vi "Launch Client Handler Actor.vi"(6 "timeout ms (5000)":i32=5000, 8 "error in (no error)":errorcluster, 9 "Remote Address":string, 10 "WebSocket Connection in":refnum<k5>, 11 "Websocket Server in":refnum<class "Websocket Server.lvclass">) -> (0 "error out":errorcluster, 3 "Websocket Server out":refnum<class "Websocket Server.lvclass">)   [LabVIEW 2016, in "Stream Mediator.lvlib" / "Websocket Server.lvclass"]
doc: "--\nCopyright © 2017 Composed SystemsI All rights reserved.\n\nAuthor: Jon McBee <jon.mcbee@composed.io>\n\nThis library is provided \"AS IS\" ,WITHOUT WARRANTIES OR\nCONDITIONS OF ANY KIND, either express or implied.\n\nComposed Systems -- composed.io\n\nStream 0.0.1.1\nJon McBee - Composed Systems\nCopyright (c) 2017, Composed Systems"
uses:
  <userlib>/Composed Systems/Stream/Mediator/Classes/Websocket Server Actor/Websocket Server/Websocket Server.lvclass
  C:/Program Files (x86)/National Instruments/LabVIEW 2016/user.lib/Composed Systems/Stream/Mediator/Classes/Mediated Actor/Mediated Actor.lvclass
  C:/Program Files (x86)/National Instruments/LabVIEW 2016/user.lib/Composed Systems/Stream/Mediator/Classes/Mediated Asynchronous Actor/Mediated Asynchronous Actor.lvclass
  <userlib>/Composed Systems/Stream/Mediator/Classes/Websocket Server Actor/Websocket Server/Websocket Server.lvclass/Websocket Server.ctl
  <userlib>/Composed Systems/Stream/Mediator/Classes/Websocket Client Handler Actor/Websocket Client Handler/Websocket Client Handler.lvclass
  <vilib>/MediaMongrels Ltd/WebSockets/WebSockets/WebSockets.lvlib
  <userlib>/Composed Systems/Stream/Mediator/Classes/Mediated Actor/Mediated Actor.lvclass
  <userlib>/Composed Systems/Stream/Mediator/Classes/Mediated Asynchronous Actor/Mediated Asynchronous Actor.lvclass
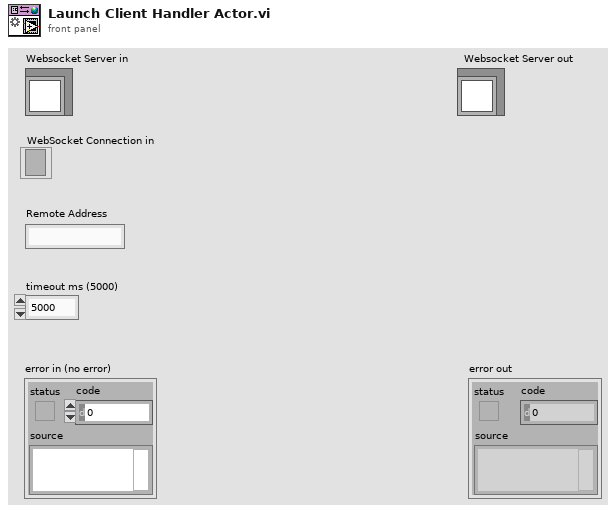
[diagram p1: front panel]
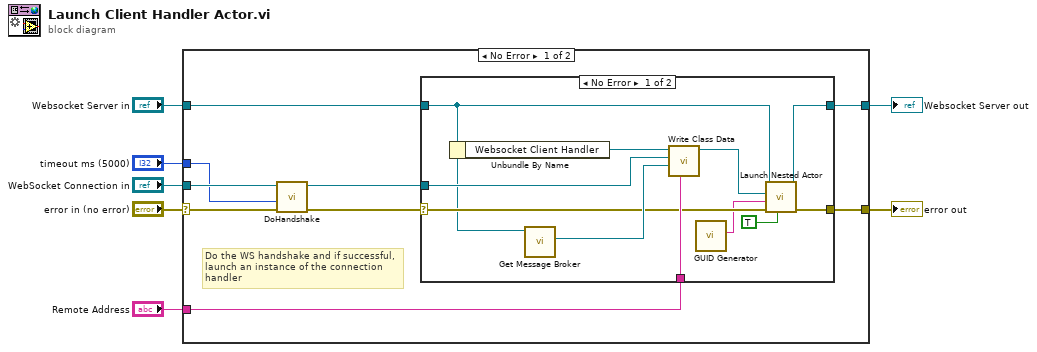
[diagram p0: block diagram]
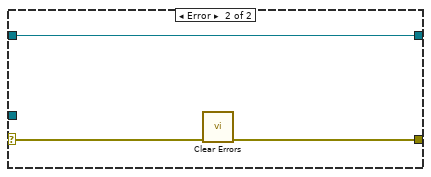
[diagram p2: hidden frame]
diagram:
  n1 = case shown="No Error" "error in (no error)" {
    selector: "error in (no error)" -> [w16 w32]
    tunnel: [w12 w32] -> w6
    tunnel: [w13 w31] -> w4
    tunnel: "Websocket Server in" -> [w9 w31]
    tunnel: "WebSocket Connection in" -> [w15 _]
    tunnel: "Remote Address" -> [w11 _]
    tunnel: "timeout ms (5000)" -> [w14 _]
    frame No Error {
      # "Do the WS handshake and if successful, launch an instance of the connection handler"
      n2 = call <vilib>:"DoHandshake.vi"("error in (no error)"=w16, "timeout ms (5000)"=w14, "WebSocket Connection in"=w15) -> ("error out"=w8:errorcluster, "WebSocket Connection out"=w10:refnum<k5>)  [unwired: 5 in, 2 out]
      n3 = case shown="No Error" w8 {
        selector: w8 -> [w23 w29]
        tunnel: [w20 w30] -> w13
        tunnel: [w22 w28] -> w12
        tunnel: w11 -> [w27 _]
        tunnel: w10 -> [w26 _]
        tunnel: w9 -> [w21 w30]
        frame No Error {
          n4 = Unbundle By Name(w21) -> ("Websocket Client Handler"=w25:refnum<class "Websocket Client Handler.lvclass">)
          n5 = call <userlib>:"Get Message Broker.vi"("Mediated Actor in"=w21) -> ("Message Broker"=w24:refnum<class "Message Broker Interface.lvclass">)  [unwired: 9 in, 1 out]
          n6 = call <userlib>:"Write Class Data.vi"("Remote Address"=w27, "Message Broker"=w24, "Connection ID"=w26, "Websocket Client Handler in"=w25) -> ("Websocket Client Handler out"=w19:refnum<class "Websocket Client Handler.lvclass">)  [unwired: 6 in, 1 out]
          n7 = call <vilib>:"GUID Generator.vi"() -> ("GUID"=w18:string)  [unwired: 10 in, 1 out]
          n8 = call <userlib>:"Launch Nested Actor.vi"("Auto Stop?"=TRUE, "error in (no error)"=w23, "Actor Name"=w18, "Nested Mediated Asynchronous Actor in"=w19, "Caller Mediated Asynchronous Actor in"=w21) -> ("error out"=w22:errorcluster, "Caller Mediated Asynchronous Actor out"=w20:refnum<class "Websocket Server.lvclass">)  [unwired: 4 in, 1 out]
        }
        frame Error {
          n9 = call <vilib>:"Clear Errors.vi"("error in (no error)"=w29) -> ("error out"=w28:errorcluster)  [unwired: 5 in, 1 out]
        }
      }
    }
    frame Error {
    }
  }
  "error out" <- w6
  "Websocket Server out" <- w4
